vi "GetFunctionGenStatus.vi"(8 "error in (no error)":errorcluster) -> (0 "error out":errorcluster, 3 "function return":i16)   [LabVIEW 2013, in "HS3OverallRoutines.lvlib"]
doc: "The TiePieSCOPE HS801, TP801 and Handyscope HS3 can\nhave a built-in arbitrary waveform generator. When this function returns E_NO_GENERATOR, the HS801, TP801 or Handyscope HS3 is equipped with a simple square wave generator.\n\nInput: -\nOutput: Return value E_NO_ERRORS | E_NO_GENERATOR | E_NO_HARDWARE\n\nshort int GetFunctionGenStatus ( void );"
uses:
  HS3OverallRoutines.lvlib
  hs3.dll
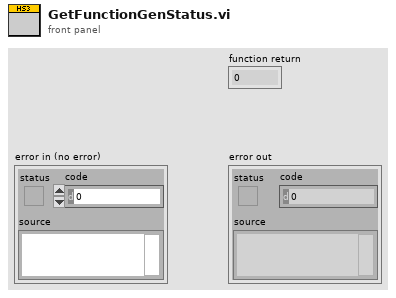
[diagram p1: front panel]
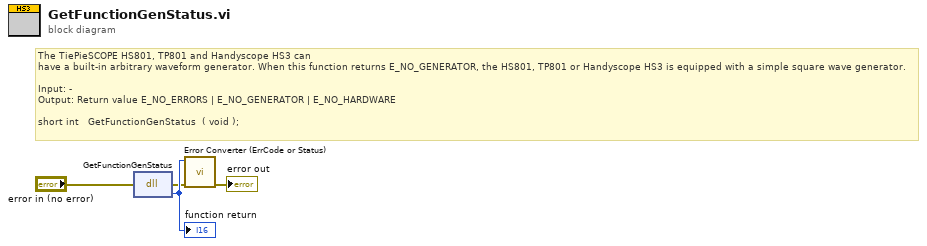
[diagram p0: block diagram]
diagram:
  # "The TiePieSCOPE HS801, TP801 and Handyscope HS3 can\nhave a built-in arbitrary waveform generator. When this function returns E_NO_GENERATOR, the HS801, TP801 or Handyscope HS3 is equipped with a simple square wave generator.\n\nInput: -\nOutput: Return value E_NO_ERRORS | E_NO_GENERATOR | E_NO_HARDWARE\n\nshort int \t\tGetFunctionGenStatus\t\t( void );"
  n1 = dll-call lib="C:/Documents and Settings/admin/Pulpit/HS3 LabViewLib/HS3_WRAPPER/OverallRoutines/hs3.*" fn="GetFunctionGenStatus"(error in="error in (no error)") -> (error out=w2:errorcluster, w4:i16)  [unwired: 2 in, 1 out]
  "function return" <- w4
  n2 = call "Error Converter (ErrCode or Status).vi"("error in (no error)"=w2, "error code"=w4) -> ("error out"=→"error out":errorcluster)  [unwired: 9 in]
